vi "IMU Get Euler Angle Landscape.vi"(8 "error in (no error)":errorcluster) -> (0 "error out":errorcluster, 2 "timestamp":i64, 3 "Euler angles":T1)   [LabVIEW 2026, in "MrcLib.lvlib"]
doc: "Returns the computed Euler angles of the built-in sensor assuming it is mounted vertically with long edge parallel to the ground (somewhat common)."
uses:
  MrcLib.lvlib
  Types/MRC Euler Angles Values.ctl
  <vilib>/MRC/MrcLib/VIs/IMU/MRC IMU Get Euler Angles Landscape.vi
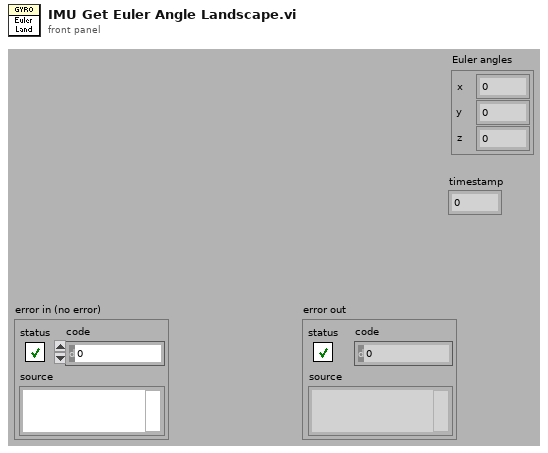
[diagram p1: front panel]
types:
  T1 = typedef "MrcLib.lvlib/MRC Euler Angles Values.ctl" = cluster{"x":dbl, "y":dbl, "z":dbl}
  T2 = typedef "MrcLib.lvlib/MRC Euler Angles.ctl" = cluster{"timestamp":i64, "x":dbl, "y":dbl, "z":dbl}
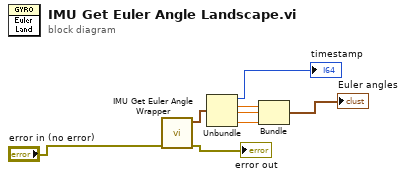
[diagram p0: block diagram]
diagram:
  n1 = call-poly "IMU Get Euler Angle Wrapper.vi"("error in (no error)"="error in (no error)") -> ("error out"=→"error out":errorcluster, "angles"=w6:T2)  [unwired: 8 in, 1 out]
  n2 = Unbundle(w6) -> ("timestamp"=→"timestamp":i64, "x"=w5:dbl, "y"=w4:dbl, "z"=w3:dbl)
  n3 = Bundle("x"=w5, "y"=w4, "z"=w3) -> (→"Euler angles":cluster{"x":dbl, "y":dbl, "z":dbl})  [unwired: 1 in]
